vi "hardware_initialize_hardware.vi"(8 "error in (no error)":errorcluster, 11 "hydraharp in":refnum<class "hydraharp.lvclass">) -> (0 "error out":errorcluster, 3 "hydraharp out":refnum<class "hydraharp.lvclass">)   [LabVIEW 2015, in "hydraharp.lvclass"]
uses:
  hydraharp.lvclass
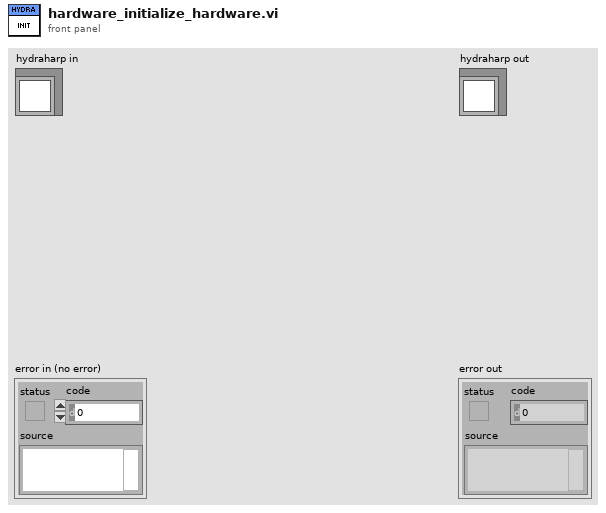
[diagram p1: front panel]
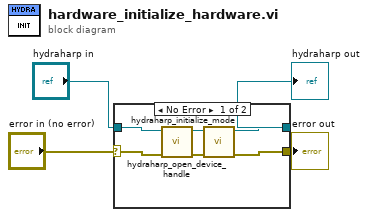
[diagram p0: block diagram]
diagram:
  n1 = case shown="No Error" "error in (no error)" {
    selector: "error in (no error)" -> [w10 w11]
    tunnel: "hydraharp in" -> [w9 w12]
    tunnel: [w6 w11] -> w2
    tunnel: [w5 w12] -> w1
    frame No Error {
      n2 = call "hydraharp_open_device_handle.vi"("error in (no error)"=w10, "hydraharp in"=w9) -> ("error out"=w8:errorcluster, "hydraharp out"=w7:refnum<class "hydraharp.lvclass">)  [unwired: 8 in]
      n3 = call "hydraharp_initialize_mode.vi"("error in (no error)"=w8, "hydraharp in"=w7) -> ("error out"=w6:errorcluster, "hydraharp out"=w5:refnum<class "hydraharp.lvclass">)  [unwired: 8 in]
    }
    frame Error {
    }
  }
  "error out" <- w2
  "hydraharp out" <- w1
